vi "SP Get Limit Data From Run Data.vi"(5 "Parameter":T1={"Stimulus Port"=1, "Response Port"=1} {"Stimulus Port" min=1 step=1; "Response Port" min=1 step=1}, 7 "Limit":T2={"Parameter"={"Stimulus Port"=1, "Response Port"=1}, "Format"=enum."Log Mag", "Limit Type"=enum."Upper", "Points"=[], "Referential Limit"={"Ref Limit"=FALSE, "Ref Type"=enum."Current", "Model"="", "Serial"="", "Run Type"=enum."Most Recent", "Run"=0, "Field"="", "Field Value"=""}, "Limit #"=1} {"Parameter"."Stimulus Port" min=1 step=1; "Parameter"."Response Port" min=1 step=1}, 8 "error in (no error)":errorcluster, 10 "Run Waveforms":waveform(dbl)[](array[waveform]), 11 "File Information":T7) -> (0 "error out":errorcluster, 1 "Data Waveform":waveform(dbl), 2 "Frequency Waveform":waveform(dbl), 3 "Found?":bool)   [LabVIEW 2011]
uses:
  TDMS/TDMS File.ctl
  TDMS/TDMS Run.ctl
  TDMS/TDMS Channel (Sxx).ctl
  typedefs/Field Record.ctl
  typedefs/Field DataTypes.ctl
  typedefs/Field NextItem.ctl
  TypeDefs/SP Limit.ctl
  TypeDefs/SP Parameter.ctl
  TypeDefs/SP Format.ctl
  TypeDefs/SP Limit Type.ctl
  TypeDefs/SP Limit Point.ctl
  Test Referential Limit.ctl
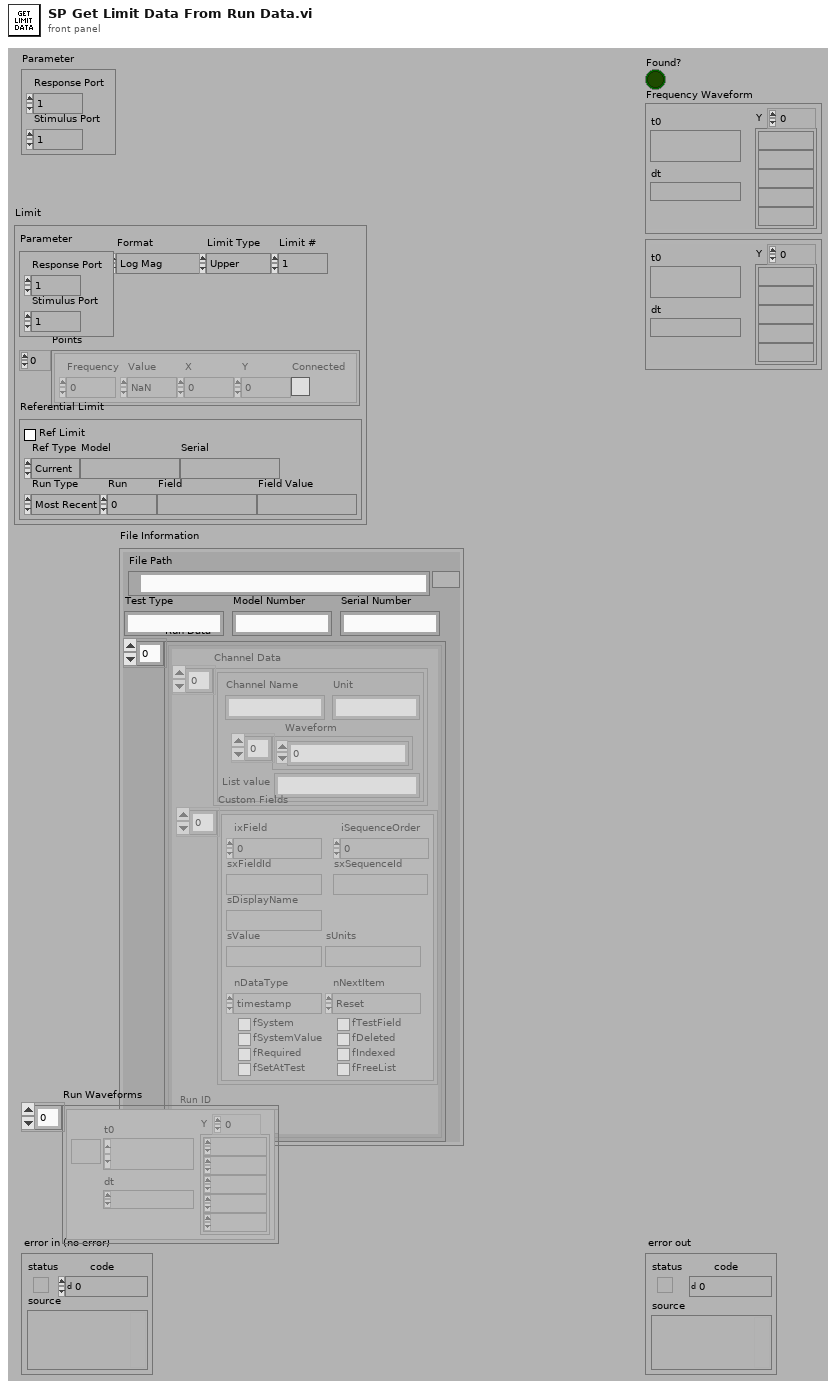
[diagram p1: front panel]
types:
  T1 = typedef "SP Parameter.ctl" = cluster{"Stimulus Port":i8, "Response Port":i8}
  T2 = typedef "SP Limit.ctl" = cluster{"Parameter":T1, "Format":T3, "Limit Type":T4, "Points":T5[], "Referential Limit":T6, "Limit #":i8}
  T3 = typedef "SP Format.ctl" = enum16{"Log Mag", "Lin Mag", "SWR", "Phase", "Expanded Phase", "Delay", "Insertion Loss", "Isolation", "Return Loss"}
  T4 = typedef "SP Limit Type.ctl" = enum16{"Upper", "Lower", "Delta", "Filter", "Referential"}
  T5 = typedef "SP Limit Point.ctl" = cluster{"Frequency":dbl, "Value":dbl, "X":dbl, "Y":dbl, "Connected":bool}
  T6 = typedef "Test Referential Limit.ctl" = cluster{"Ref Limit":bool, "Ref Type":enum16{"Current", "Specify"}, "Model":string, "Serial":string, "Run Type":enum16{"Most Recent", "Run #", "Match Field"}, "Run":i32, "Field":string, "Field Value":string}
  T7 = typedef "TDMS File.ctl" = cluster{"File Path":path, "Run Data":T8[], "Serial Number":string, "Model Number":string, "Test Type":string}
  T8 = typedef "TDMS Run.ctl" = cluster{"Channel Data":T9[], "Custom Fields":T10[], "Run ID":string}
  T9 = typedef "TDMS Channel (Sxx).ctl" = cluster{"Channel Name":string, "Waveform":dbl[], "Unit":string, "List value":string}
  T10 = typedef "Field Record.ctl" = cluster{"ixField":i32, "iSequenceOrder":i32, "sxFieldId":string, "sxSequenceId":string, "sDisplayName":string, "sValue":string, "sUnits":string, "nDataType":T11, "nNextItem":T12, "fSystem":bool, "fSystemValue":bool, "fRequired":bool, "fSetAtTest":bool, "fTestField":bool, "fDeleted":bool, "fIndexed":bool, "fFreeList":bool}
  T11 = typedef "Field DataTypes.ctl" = enum32{"text", "numeric", "list", "timestamp", "boolean"}
  T12 = typedef "Field NextItem.ctl" = enum32{"Reset", "Retain", "Auto-Increment"}
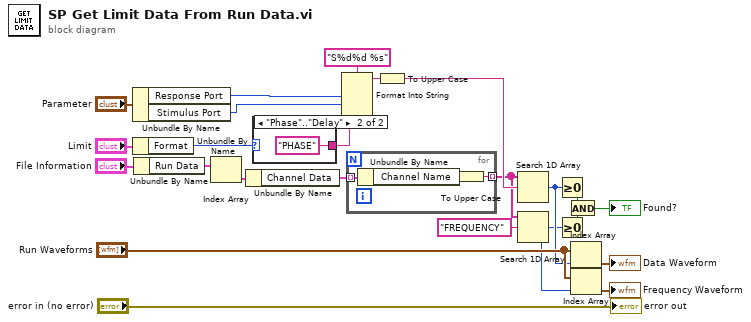
[diagram p0: block diagram]
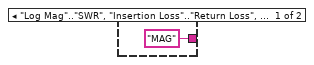
[diagram p2: hidden frame]
diagram:
  n1 = Unbundle By Name("Parameter") -> ("Response Port"=w2:i8, "Stimulus Port"=w1:i8)
  n2 = Unbundle By Name("Limit") -> ("Format"=w20:T3)
  n3 = Unbundle By Name("File Information") -> ("Run Data"=w18:T8[])
  n4 = Index Array(array=w18) -> (element=w19:T8)  [unwired: 1 in]
  n5 = Unbundle By Name(w19) -> ("Channel Data"=w16:T9[])
  n6 = case shown="\"Phase\"..\"Delay\"" w20 {
    tunnel: ["MAG" ("format string") "PHASE" ("format string")] -> w13
    frame "Log Mag".."SWR", "Insertion Loss".."Return Loss", Default {
    }
    frame "Phase".."Delay" {
    }
  }
  n7 = Format Into String(format string="S%d%d %s", w2, w1, w13) -> (resulting string=w21:string)  [unwired: 2 in, 1 out]
  n8 = for {
    tunnel: w16 -> [w29] mode=indexing
    tunnel: [w27] -> w11 mode=indexing
    n9 = Unbundle By Name(w29) -> ("Channel Name"=w28:string)
    n10 = To Upper Case(1:w28) -> (0:w27:string)
  }
  n11 = To Upper Case(1:w21) -> (0:w12:string)
  n12 = Search 1D Array(1D array=w11, element=w12) -> (index of element=w5:i32)  [unwired: 1 out]
  n13 = Search 1D Array(1D array=w11, element="FREQUENCY") -> (index of element=w4:i32)  [unwired: 1 out]
  n14 = Greater Or Equal To 0?(x=w5) -> (x >= 0?=w14:bool)
  n15 = Greater Or Equal To 0?(x=w4) -> (x >= 0?=w15:bool)
  n16 = And(x=w14, y=w15) -> (x .and. y?=→"Found?":bool)
  n17 = Index Array(array="Run Waveforms", index=w5) -> (element=→"Data Waveform":waveform(dbl))
  n18 = Index Array(array="Run Waveforms", index=w4) -> (element=→"Frequency Waveform":waveform(dbl))
  "error out" <- "error in (no error)"
